vi "Get Parameter.vi"(7 "file level":T1, 8 "error in":errorcluster, 9 "Parameter Name":string, 10 "data type":T2, 11 "TDMS in":refnum<class "TDMS.lvclass">) -> (0 "error out":errorcluster, 1 "found?":bool, 2 "parameter":variant, 3 "TDMS out":refnum<class "TDMS.lvclass">)   [LabVIEW 2011, in "TDMS.lvclass"]
uses:
  TDMS.lvclass
  Parameter Data Type.ctl
  File Level.ctl
  TDMS.lvclass/TDMS.ctl
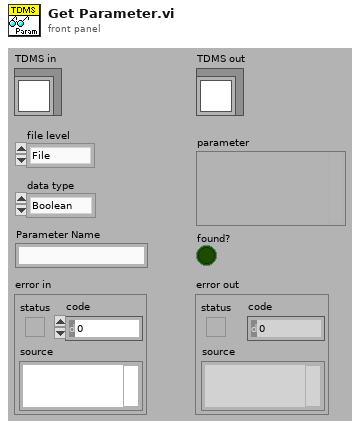
[diagram p1: front panel]
types:
  T1 = typedef "TDMS.lvclass/File Level.ctl" = enum16{"File", "Group", "Channel"}
  T2 = typedef "TDMS.lvclass/Parameter Data Type.ctl" = enum16{"Boolean", "U32", "I32", "Double", "String", "Path"}
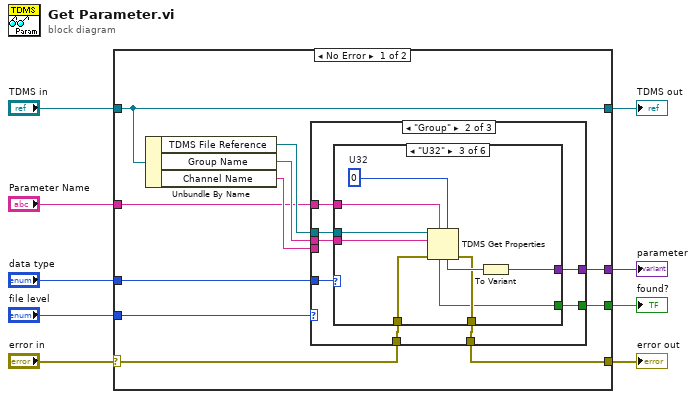
[diagram p0: block diagram]
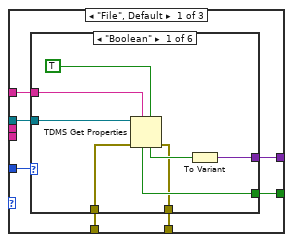
[diagram p2: hidden frame]
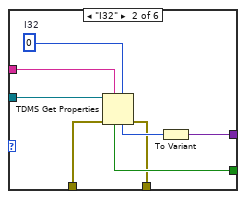
[diagram p3: hidden frame]
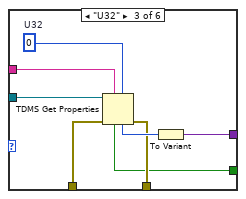
[diagram p4: hidden frame]
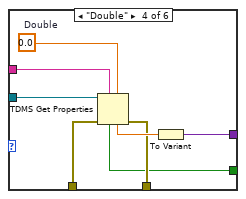
[diagram p5: hidden frame]
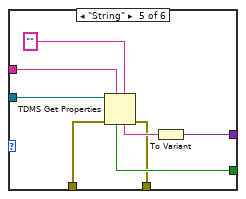
[diagram p6: hidden frame]
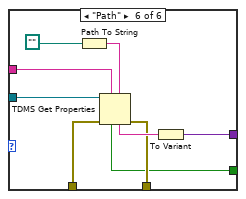
[diagram p7: hidden frame]
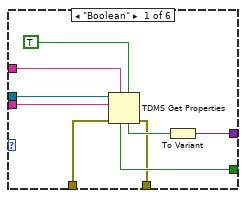
[diagram p8: hidden frame]
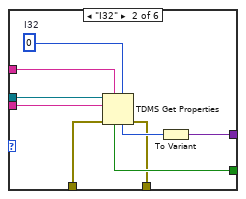
[diagram p9: hidden frame]
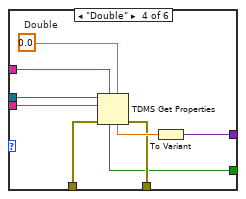
[diagram p10: hidden frame]
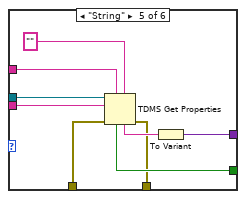
[diagram p11: hidden frame]
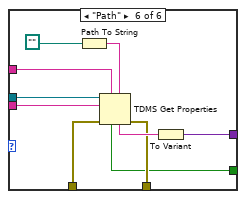
[diagram p12: hidden frame]
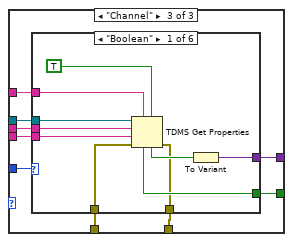
[diagram p13: hidden frame]
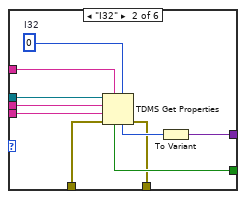
[diagram p14: hidden frame]
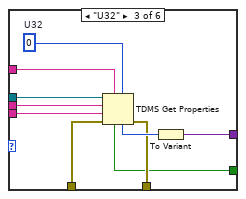
[diagram p15: hidden frame]
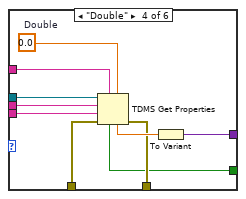
[diagram p16: hidden frame]
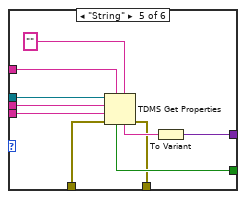
[diagram p17: hidden frame]
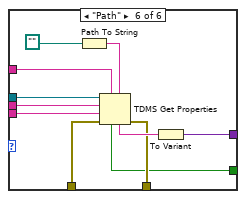
[diagram p18: hidden frame]
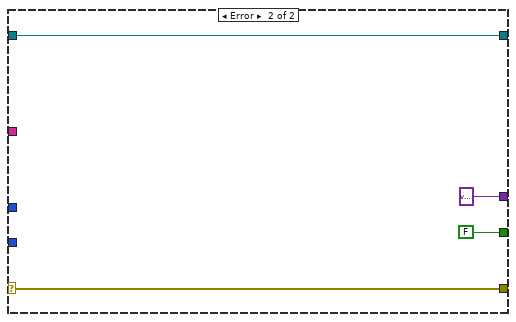
[diagram p19: hidden frame]
diagram:
  n1 = case shown="No Error" "error in" {
    selector: "error in" -> [w17 w212]
    tunnel: [w16 w212] -> w8
    tunnel: [w20 w213] -> w6
    tunnel: "TDMS in" -> [w20 w213]
    tunnel: "Parameter Name" -> [w14 _]
    tunnel: "data type" -> [w13 _]
    tunnel: "file level" -> [w12 _]
    tunnel: [w11 variant ("Variant")] -> w2
    tunnel: [w10 FALSE] -> w1
    frame No Error {
      n2 = Unbundle By Name(w20) -> ("TDMS File Reference"=w19:refnum<k34>, "Group Name"=w18:string, "Channel Name"=w15:string)
      n3 = case shown="\"Group\"" w12 {
        tunnel: [w27 w84 w142] -> w11
        tunnel: w19 -> [w23 w83 w147]
        tunnel: w18 -> [_ w82 w146]
        tunnel: w13 -> [w24 w81 w140]
        tunnel: w17 -> [w22 w80 w144]
        tunnel: [w26 w79 w141] -> w10
        tunnel: [w21 w78 w143] -> w16
        tunnel: w14 -> [w25 w77 w148]
        tunnel: w15 -> [_ _ w145]
        frame "File", Default {
          n4 = case shown="\"Boolean\"" w24 {
            tunnel: w23 -> [w35 w43 w51 w59 w67 w76]
            tunnel: [w32 w41 w49 w57 w65 w74] -> w27
            tunnel: w22 -> [w31 w37 w46 w54 w61 w71]
            tunnel: [w30 w38 w44 w52 w62 w68] -> w26
            tunnel: [w29 w36 w45 w53 w60 w70] -> w21
            tunnel: w25 -> [w28 w39 w47 w55 w63 w69]
            frame "Boolean" {
              n5 = TDMS Get Properties(5:TRUE, 7:w28, 8:w31, 11:w35) -> (0:w29:errorcluster, 4:w33:bool, 6:w30:bool)  [unwired: 2 in, 3 out]
              n6 = To Variant(anything=w33) -> (Variant=w32:variant)
            }
            frame "I32" {
              w40 = 0  # I32
              n7 = TDMS Get Properties(5:w40, 7:w39, 8:w37, 11:w43) -> (0:w36:errorcluster, 4:w42:i32, 6:w38:bool)  [unwired: 2 in, 3 out]
              n8 = To Variant(anything=w42) -> (Variant=w41:variant)
            }
            frame "U32" {
              w48 = 0  # U32
              n9 = TDMS Get Properties(5:w48, 7:w47, 8:w46, 11:w51) -> (0:w45:errorcluster, 4:w50:i32, 6:w44:bool)  [unwired: 2 in, 3 out]
              n10 = To Variant(anything=w50) -> (Variant=w49:variant)
            }
            frame "Double" {
              w56 = 0.0  # Double
              n11 = TDMS Get Properties(5:w56, 7:w55, 8:w54, 11:w59) -> (0:w53:errorcluster, 4:w58:dbl, 6:w52:bool)  [unwired: 2 in, 3 out]
              n12 = To Variant(anything=w58) -> (Variant=w57:variant)
            }
            frame "String" {
              n13 = TDMS Get Properties(5:"", 7:w63, 8:w61, 11:w67) -> (0:w60:errorcluster, 4:w66:string, 6:w62:bool)  [unwired: 2 in, 3 out]
              n14 = To Variant(anything=w66) -> (Variant=w65:variant)
            }
            frame "Path" {
              n15 = Path To String(path=path "") -> (string=w72:string)
              n16 = TDMS Get Properties(5:w72, 7:w69, 8:w71, 11:w76) -> (0:w70:errorcluster, 4:w75:string, 6:w68:bool)  [unwired: 2 in, 3 out]
              n17 = To Variant(anything=w75) -> (Variant=w74:variant)
            }
          }
        }
        frame "Group" {
          n18 = case shown="\"U32\"" w81 {
            tunnel: w83 -> [w93 w102 w111 w120 w129 w139]
            tunnel: w82 -> [w92 w101 w110 w119 w128 w138]
            tunnel: [w89 w99 w108 w117 w126 w136] -> w84
            tunnel: w80 -> [w88 w95 w105 w114 w122 w133]
            tunnel: [w87 w96 w103 w112 w123 w130] -> w79
            tunnel: [w86 w94 w104 w113 w121 w132] -> w78
            tunnel: w77 -> [w85 w97 w106 w115 w124 w131]
            frame "Boolean" {
              n19 = TDMS Get Properties(5:TRUE, 7:w85, 8:w88, 10:w92, 11:w93) -> (0:w86:errorcluster, 4:w90:bool, 6:w87:bool)  [unwired: 1 in, 3 out]
              n20 = To Variant(anything=w90) -> (Variant=w89:variant)
            }
            frame "I32" {
              w98 = 0  # I32
              n21 = TDMS Get Properties(5:w98, 7:w97, 8:w95, 10:w101, 11:w102) -> (0:w94:errorcluster, 4:w100:i32, 6:w96:bool)  [unwired: 1 in, 3 out]
              n22 = To Variant(anything=w100) -> (Variant=w99:variant)
            }
            frame "U32" {
              w107 = 0  # U32
              n23 = TDMS Get Properties(5:w107, 7:w106, 8:w105, 10:w110, 11:w111) -> (0:w104:errorcluster, 4:w109:i32, 6:w103:bool)  [unwired: 1 in, 3 out]
              n24 = To Variant(anything=w109) -> (Variant=w108:variant)
            }
            frame "Double" {
              w116 = 0.0  # Double
              n25 = TDMS Get Properties(5:w116, 7:w115, 8:w114, 10:w119, 11:w120) -> (0:w113:errorcluster, 4:w118:dbl, 6:w112:bool)  [unwired: 1 in, 3 out]
              n26 = To Variant(anything=w118) -> (Variant=w117:variant)
            }
            frame "String" {
              n27 = TDMS Get Properties(5:"", 7:w124, 8:w122, 10:w128, 11:w129) -> (0:w121:errorcluster, 4:w127:string, 6:w123:bool)  [unwired: 1 in, 3 out]
              n28 = To Variant(anything=w127) -> (Variant=w126:variant)
            }
            frame "Path" {
              n29 = Path To String(path=path "") -> (string=w134:string)
              n30 = TDMS Get Properties(5:w134, 7:w131, 8:w133, 10:w138, 11:w139) -> (0:w132:errorcluster, 4:w137:string, 6:w130:bool)  [unwired: 1 in, 3 out]
              n31 = To Variant(anything=w137) -> (Variant=w136:variant)
            }
          }
        }
        frame "Channel" {
          n32 = case shown="\"Boolean\"" w140 {
            tunnel: w147 -> [w158 w168 w178 w188 w198 w209]
            tunnel: w146 -> [w157 w167 w177 w187 w197 w208]
            tunnel: [w154 w165 w175 w185 w195 w206] -> w142
            tunnel: w144 -> [w153 w161 w172 w182 w191 w203]
            tunnel: [w152 w162 w170 w180 w192 w200] -> w141
            tunnel: [w151 w160 w171 w181 w190 w202] -> w143
            tunnel: w148 -> [w150 w163 w173 w183 w193 w201]
            tunnel: w145 -> [w149 w159 w169 w179 w189 w199]
            frame "Boolean" {
              n33 = TDMS Get Properties(5:TRUE, 7:w150, 8:w153, 9:w149, 10:w157, 11:w158) -> (0:w151:errorcluster, 4:w155:bool, 6:w152:bool)  [unwired: 3 out]
              n34 = To Variant(anything=w155) -> (Variant=w154:variant)
            }
            frame "I32" {
              w164 = 0  # I32
              n35 = TDMS Get Properties(5:w164, 7:w163, 8:w161, 9:w159, 10:w167, 11:w168) -> (0:w160:errorcluster, 4:w166:i32, 6:w162:bool)  [unwired: 3 out]
              n36 = To Variant(anything=w166) -> (Variant=w165:variant)
            }
            frame "U32" {
              w174 = 0  # U32
              n37 = TDMS Get Properties(5:w174, 7:w173, 8:w172, 9:w169, 10:w177, 11:w178) -> (0:w171:errorcluster, 4:w176:i32, 6:w170:bool)  [unwired: 3 out]
              n38 = To Variant(anything=w176) -> (Variant=w175:variant)
            }
            frame "Double" {
              w184 = 0.0  # Double
              n39 = TDMS Get Properties(5:w184, 7:w183, 8:w182, 9:w179, 10:w187, 11:w188) -> (0:w181:errorcluster, 4:w186:dbl, 6:w180:bool)  [unwired: 3 out]
              n40 = To Variant(anything=w186) -> (Variant=w185:variant)
            }
            frame "String" {
              n41 = TDMS Get Properties(5:"", 7:w193, 8:w191, 9:w189, 10:w197, 11:w198) -> (0:w190:errorcluster, 4:w196:string, 6:w192:bool)  [unwired: 3 out]
              n42 = To Variant(anything=w196) -> (Variant=w195:variant)
            }
            frame "Path" {
              n43 = Path To String(path=path "") -> (string=w204:string)
              n44 = TDMS Get Properties(5:w204, 7:w201, 8:w203, 9:w199, 10:w208, 11:w209) -> (0:w202:errorcluster, 4:w207:string, 6:w200:bool)  [unwired: 3 out]
              n45 = To Variant(anything=w207) -> (Variant=w206:variant)
            }
          }
        }
      }
    }
    frame Error {
    }
  }
  "error out" <- w8
  "TDMS out" <- w6
  "parameter" <- w2
  "found?" <- w1
